vi "connect.vi"(8 "error in (no error)":errorcluster, 9 "sin6_port":dbl, 10 "sin6_addr":string, 11 "tcp socket fd":i32) -> (0 "error out":errorcluster, 3 "success":u16)   [LabVIEW 2015]
panel:
  in  "sin6_flowinto":dbl
  in  "sin6_family":string
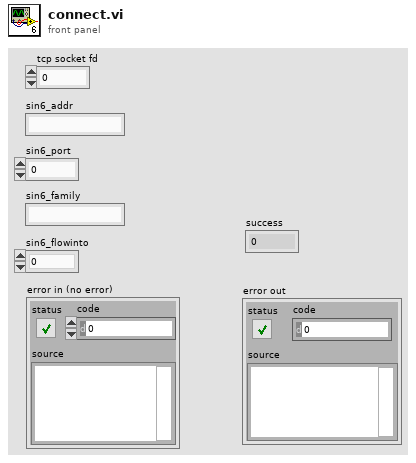
[diagram p1: front panel]
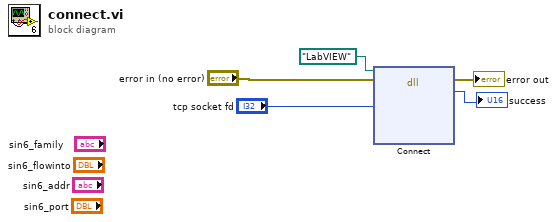
[diagram p0: block diagram]
diagram:
  n1 = dll-call lib="LabVIEW" fn="Connect"(path in=path "LabVIEW", error in="error in (no error)", "sockfd"="tcp socket fd") -> (error out=→"error out":errorcluster, "success"=→"success":u16, "sockaddr"=w1:void[])  [unwired: 5 in, 1 out]
